vi "Destroy.vi"(0 "object in":refnum<class "HPS-17000-PowerModule.lvclass">, 11 "Error In":errorcluster) -> (4 "object out":refnum<class "HPS-17000-PowerModule.lvclass">, 15 "Error Out":errorcluster)   [LabVIEW 2023, in "HPS-17000-PowerModule.lvlib" / "HPS-17000-PowerModule.lvclass"]
uses:
  HPS-17000-PowerModule.lvclass
  HPS-17000-PowerModule.lvclass/HPS-17000-PowerModule.ctl
  <vilib>/addons/_JKI.lib/Serialization/JSON/JKI JSON Serialization.lvlib
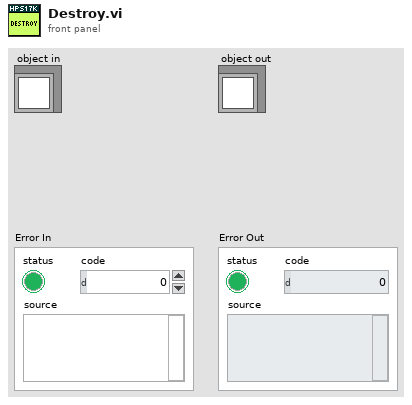
[diagram p1: front panel]
types:
  T1 = typedef "HPS-17000-PowerModule.lvlib/HPS-17000-PowerModule.lvclass/ObjectAttributes.ctl" = cluster{"JSON Config Path":path, "Configuration":T2, "GM ID":string, "HPS17000 Refs":refnum<class "HPS-17000.lvclass">[], "Stream Queues":refnum<queue>[], "connected":bool, "reserved":bool, "events":T4, "nibatterycycler_grpc_Setpoint":T5, "last timestamp":i64, "mode":T6, "range":T7}
  T2 = typedef "HPS-17000-PowerModule.lvlib/HPS-17000-PowerModule.lvclass/Configuration.ctl" = cluster{"TSN NIC IP Address":string, "HPS17000 IP Addresses":string[], "HPS Topology":enum16{"SINGLE", "MULTI"}, "Setpoint Stream Config":T3}
  T3 = typedef "Cycler.lvclass/Setpoint Stream Basic Config.ctl" = cluster{"local address":string, "receiver port":u16}
  T4 = typedef "HPS-17000.lvclass/Multi-Cycler Events.ctl" = cluster{"heartbeats events":refnum<user-event>[], "faults events":refnum<user-event>[], "network sync event":refnum<user-event>[], "setpoint status event":refnum<user-event>[]}
  T5 = typedef "NI_BC_client.lvlib/nibatterycycler_grpc_Setpoint.ctl" = cluster{"voltage":sgl, "current":sgl, "min_power":sgl, "max_power":sgl, "resistance":sgl}
  T6 = typedef "HPS-17000-PowerModule.lvlib/HPS-17000-PowerModule.lvclass/Mode.ctl" = u16
  T7 = typedef "PowerModuleInterface.lvlibp/PowerModuleInterface.lvclass/Range.ctl" = cluster{"Current Max (A)":dbl, "Current Min (A)":dbl, "Voltage Max (V)":dbl, "Voltage Min (V)":dbl}
  T8 = enum16{"open", "replace", "create", "open or create", "replace or create", "replace or create with confirmation"}
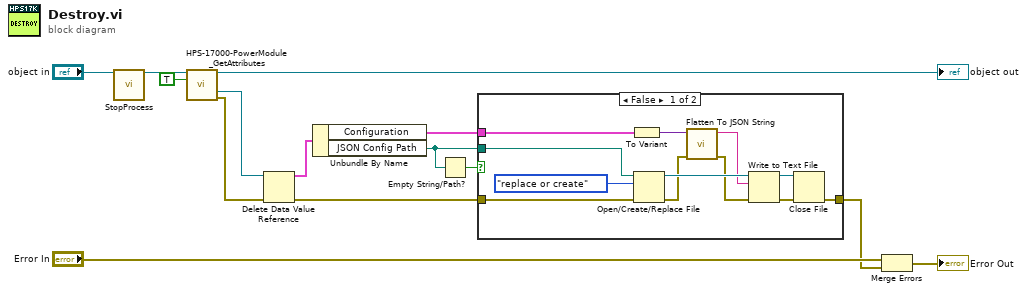
[diagram p0: block diagram]
diagram:
  n1 = call "StopProcess.vi"("reference in"="object in") -> ("reference out"=w11:refnum<class "HPS-17000-PowerModule.lvclass">)  [unwired: 17 in, 1 out]
  n2 = call "HPS-17000-PowerModule_GetAttributes.vi"("reference in"=w11, "OnlyGetDvrReference(False)"=TRUE) -> ("reference out"=→"object out":refnum<class "HPS-17000-PowerModule.lvclass">, "DataRef"=w8:refnum<data-value>, "Error Out"=w9:errorcluster)  [unwired: 10 in, 1 out]
  n3 = Delete Data Value Reference(data value reference=w8, error in=w9) -> (data value=w6:T1, error out=w5:errorcluster)
  n4 = Unbundle By Name(w6) -> ("Configuration"=w4:T2, "JSON Config Path"=w2:path)
  n5 = Empty String/Path?(string/path=w2) -> (empty?=w1:bool)
  n6 = case shown="False" w1 {
    tunnel: w5 -> [w25 w27]
    tunnel: w4 -> [w21 _]
    tunnel: [w16 w27] -> w3
    tunnel: w2 -> [w15 _]
    frame False {
      n7 = To Variant(anything=w21) -> (Variant=w20:variant)
      n8 = Open/Create/Replace File(file path (use dialog)=w15, error in=w25, operation (0:open)=T8."replace or create") -> (refnum out=w24:refnum<file>, error out=w23:errorcluster)  [unwired: 3 in, 1 out]
      n9 = call <vilib>:"Flatten To JSON String.vi"("error in"=w23, "Variant"=w20) -> ("error out"=w22:errorcluster, "JSON String"=w19:string)  [unwired: 8 in]
      n10 = Write to Text File(file (use dialog)=w24, text=w19, error in=w22) -> (refnum out=w17:refnum<file>, error out=w18:errorcluster)  [unwired: 1 in, 1 out]
      n11 = Close File(refnum=w17, error in=w18) -> (error out=w16:errorcluster)  [unwired: 1 out]
    }
    frame True {
    }
  }
  n12 = Merge Errors("Error In", w3) -> (→"Error Out":errorcluster)
